vi "HW_GEN - Search for the Parameters According to Name.vi"(7 "ParaName":string, 10 "ParaNames[]":string[](array[string]), 11 "Paravalues[] in":string[][](array[string])) -> (3 "Paravalues[] out":string[](array[string]))   [LabVIEW 2016]
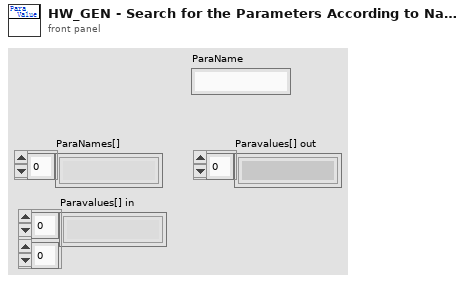
[diagram p1: front panel]
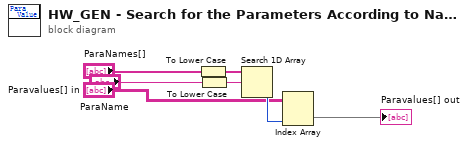
[diagram p0: block diagram]
diagram:
  n1 = To Lower Case(string="ParaNames[]") -> (all lower case string=w2:string[])
  n2 = To Lower Case(string="ParaName") -> (all lower case string=w7:string)
  n3 = Search 1D Array(1D array=w2, element=w7) -> (index of element=w5:i32)  [unwired: 1 in]
  n4 = Index Array(array="Paravalues[] in", index (col)=w5) -> (element=→"Paravalues[] out":string[])  [unwired: 1 in]
